vi "createEvents.vi"() -> (0 "error out":errorcluster, 3 "TCPComEvents out":refnum<class "TCPComEvents.lvclass">)   [LabVIEW 2016]
uses:
  TCPComEvents/TCPComEvents.lvclass
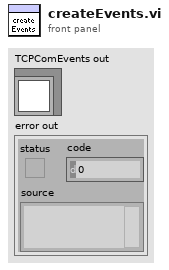
[diagram p1: front panel]
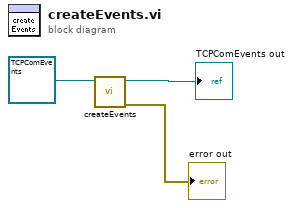
[diagram p0: block diagram]
diagram:
  n1 = call "createEvents.vi"("TCPComEvents in"=refnum<class "TCPComEvents.lvclass"> refnum ("TCPComEvents.lvclass")) -> ("error out"=→"error out":errorcluster, "TCPComEvents out"=→"TCPComEvents out":refnum<class "TCPComEvents.lvclass">)  [unwired: 9 in]
